vi "信息采集.vi"() -> (11 "Boolean":bool)   [LabVIEW 2023]
uses:
  <vilib>/sound2/lvsound2.llb/Sampling Mode.ctl
  <vilib>/sound2/lvsound2.llb/Sound Data Format.ctl
  <vilib>/sound2/lvsound2.llb/Sound Input Read (DBL).vi
panel:
  in  "退出信息采集":bool
  in  "Tab Control":enum32{"语音文字录入", "图片录入"}(tab)
  out "时间":string
  in  "保存语音文字信息":bool
  in  "开始录入语音":bool
  in  "停止录入语音":bool
  out "语音录入波形":waveform(dbl)[](graph)
  out "采集语音录入时间":string
  in  "Cluster":T1
  in  "图片录入":bool
  out "图片显示":picture
  # "个人信息采集"
  # "个人信息采集"
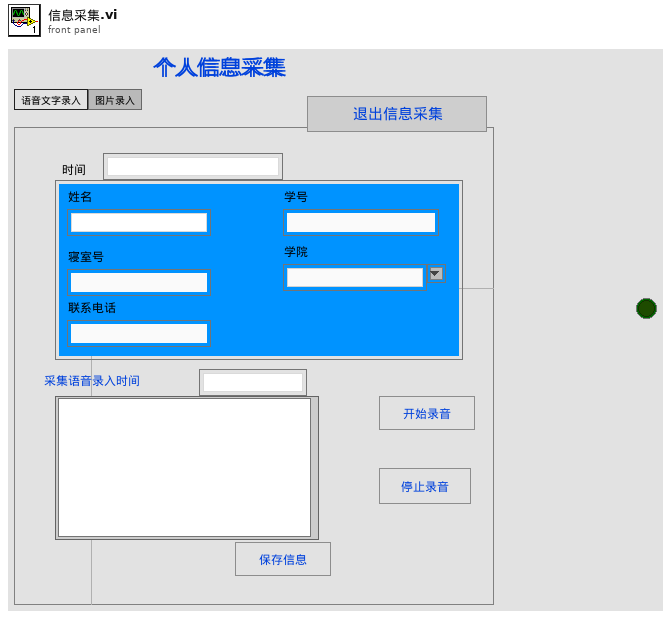
[diagram p1: front panel]
types:
  T1 = cluster{"学号":string, "姓名":string, "寝室号":string, "学院":string, "联系电话":string}
  T2 = typedef "Sound Data Format.ctl" = cluster{"sample rate (S/s)":dbl, "number of channels":i32, "bits per sample":i32}
  T3 = enum16{"open", "replace", "create", "open or create", "replace or create", "replace or create with confirmation"}
  T4 = typedef "Sampling Mode.ctl" = i32
  T5 = typedef "Sound Input Task ID.ctl" = u32
  T6 = typedef "imagedata.ctl" = cluster{"image type":i32, "image depth":i32, "image":u8[], "mask":u8[], "colors":u32[], "Rectangle":cluster{"left":i16, "top":i16, "right":i16, "bottom":i16}}
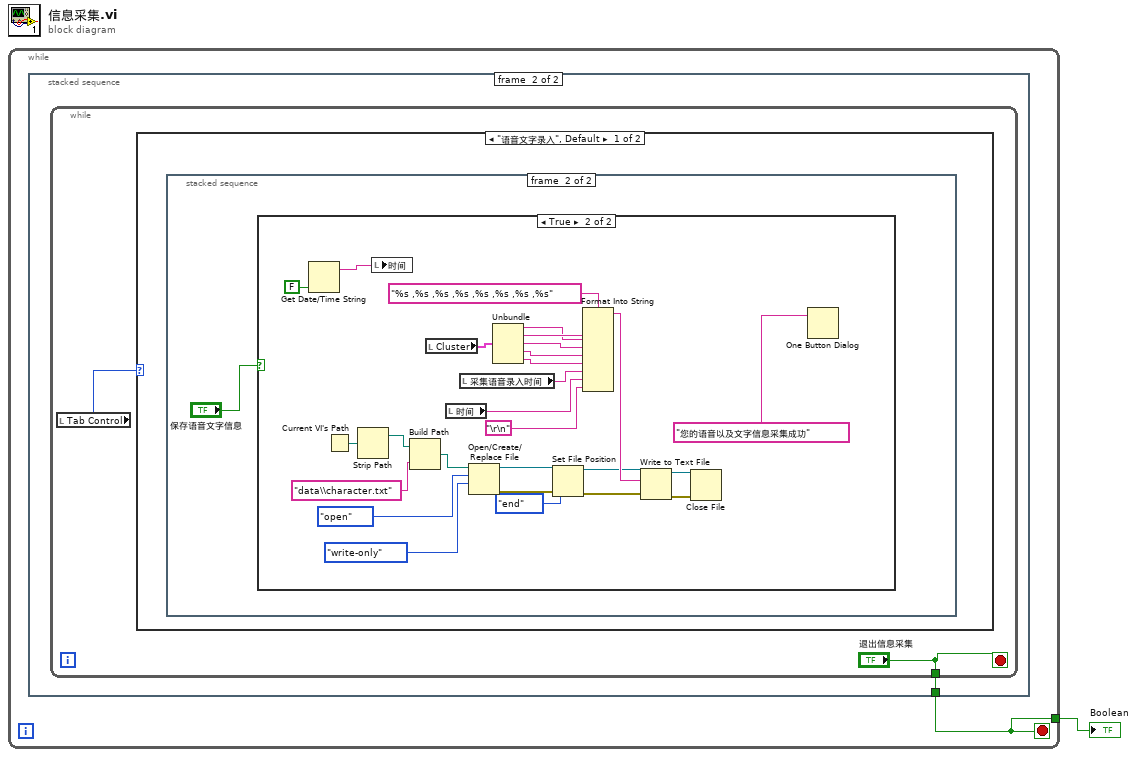
[diagram p0: block diagram]
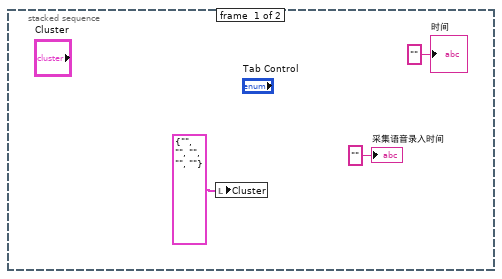
[diagram p2: hidden frame]
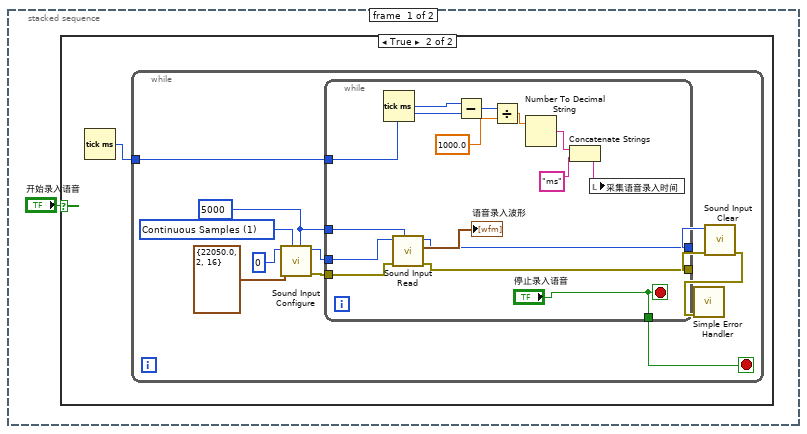
[diagram p3: hidden frame]
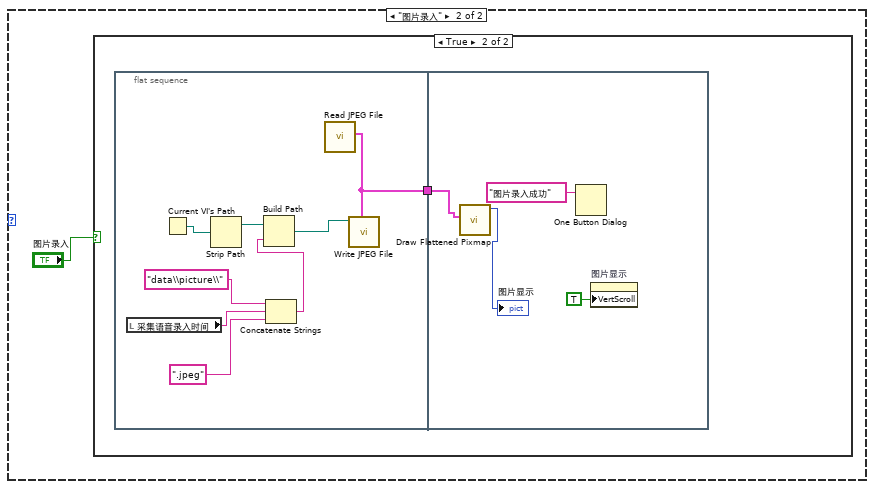
[diagram p6: hidden frame]
diagram:
  n1 = while {
    tunnel: [w2] -> w1
    stop <- w2 stop-if-true
    n2 = stacked-sequence {
      tunnel: [_ w6] -> w2
      frame #0 {
        n3 = local write "Cluster"(T1 {"学号"="", "姓名"="", "寝室号"="", "学院"="", "联系电话"=""} ("Cluster")) -> ()
        "时间" <- "" ("录入时间")
        "采集语音录入时间" <- "" ("语音录入时间")
      }
      frame #1 {
        n4 = while {
          tunnel: ["退出信息采集"] -> w6
          stop <- "退出信息采集" stop-if-true
          n5 = local read "Tab Control"() -> (w8:enum32{"语音文字录入", "图片录入"})
          n6 = case shown="\"语音文字录入\", Default" w8 {
            frame "语音文字录入", Default {
              n7 = stacked-sequence {
                frame #0 {
                  n8 = case shown="True" "开始录入语音" {
                    frame False {
                    }
                    frame True {
                      n9 = Tick Count (ms)() -> (millisecond timer value=w10:u32)
                      n10 = while {
                        tunnel: w10 -> [w12]
                        stop <- w11 stop-if-true
                        w19 = 5000 ("number of samples/ch")
                        w21 = T4 1 items=["Finite Samples", "Continuous Samples"] ("sample mode")
                        n11 = call <vilib>:"Sound Input Configure.vi"("number of samples/ch"=w19, "sample mode"=w21, "sound format"=T2 {"sample rate (S/s)"=22050.0, "number of channels"=2, "bits per sample"=16}, "device ID"=u32 0) -> ("error out"=w16:errorcluster, "task ID"=w17:T5)  [unwired: 6 in]
                        n12 = while {
                          tunnel: w19 -> [w36]
                          tunnel: w17 -> [w35]
                          tunnel: w16 -> [w34]
                          tunnel: [w32] -> w15
                          tunnel: [w31] -> w14
                          tunnel: w12 -> [w29]
                          tunnel: ["停止录入语音"] -> w11
                          stop <- "停止录入语音" stop-if-true
                          n13 = Tick Count (ms)() -> (millisecond timer value=w30:u32)
                          n14 = call-poly <vilib>:"Sound Input Read.vi"("number of samples/ch"=w36, "error in (no error)"=w34, "task ID"=w35) -> ("error out"=w31:errorcluster, "data"=→"语音录入波形":waveform(dbl)[], "task ID out"=w32:T5)  [unwired: 6 in]
                          n15 = Subtract(x=w30, y=w29) -> (x-y=w27:u32)
                          n16 = Divide(x=w27, y=1000.0) -> (x/y=w26:dbl)
                          n17 = Number To Decimal String(number=w26) -> (decimal integer string=w25:string)  [unwired: 1 in]
                          n18 = Concatenate Strings(w25, "ms" ("string")) -> (w23:string)
                          n19 = local write "采集语音录入时间"(w23) -> ()
                        }
                        n20 = call <vilib>:"Sound Input Clear.vi"("error in (no error)"=w14, "task ID"=w15) -> ("error out"=w13:errorcluster)  [unwired: 9 in]
                        n21 = call <vilib>:"Simple Error Handler.vi"("error in (no error)"=w13) -> ()  [unwired: 4 in, 5 out]
                      }
                    }
                  }
                }
                frame #1 {
                  n22 = case shown="True" "保存语音文字信息" {
                    frame False {
                    }
                    frame True {
                      n23 = Get Date/Time String(want seconds? (F)=FALSE) -> (date string=w56:string)  [unwired: 2 in, 1 out]
                      n24 = Current VI's Path() -> (path=w55:path)
                      n25 = Strip Path(path=w55) -> (stripped path=w54:path)  [unwired: 1 out]
                      n26 = local write "时间"(w56) -> ()
                      n27 = Build Path(base path=w54, name or relative path="data\\character.txt") -> (appended path=w50:path)
                      n28 = local read "Cluster"() -> (w64:T1)
                      n29 = local read "时间"() -> (w52:string)
                      n30 = local read "采集语音录入时间"() -> (w53:string)
                      n31 = Open/Create/Replace File(file path (use dialog)=w50, operation (0:open)=T3."open", access (0:read/write)=enum16{"read/write", "read-only", "write-only"}."write-only") -> (refnum out=w42:refnum<file>, error out=w40:errorcluster)  [unwired: 3 in, 1 out]
                      n32 = Unbundle(w64) -> ("学号"=w61:string, "姓名"=w62:string, "寝室号"=w60:string, "学院"=w59:string, "联系电话"=w58:string)
                      n33 = Set File Position(refnum=w42, from (0:start)=enum16{"start", "end", "current"}."end", error in=w40) -> (refnum out=w41:refnum<file>, error out=w39:errorcluster)  [unwired: 1 in]
                      n34 = Format Into String(format string="%s ,%s ,%s ,%s ,%s ,%s ,%s ,%s", w62, w61, w60, w59, w58, w53, w52, "\r\n") -> (resulting string=w46:string)  [unwired: 2 in, 1 out]
                      n35 = Write to Text File(file (use dialog)=w41, text=w46, error in=w39) -> (refnum out=w44:refnum<file>, error out=w45:errorcluster)  [unwired: 1 in, 1 out]
                      n36 = Close File(refnum=w44, error in=w45) -> ()  [unwired: 2 out]
                      n37 = One Button Dialog(message="您的语音以及文字信息采集成功") -> ()  [unwired: 1 in, 1 out]
                    }
                  }
                }
              }
            }
            frame "图片录入" {
              n38 = case shown="True" "图片录入" {
                frame False {
                }
                frame True {
                  n39 = flat-sequence {
                    tunnel: [w67] -> w66
                    tunnel: w66 -> [w78]
                    frame #0 {
                      n40 = local read "采集语音录入时间"() -> (w70:string)
                      n41 = Current VI's Path() -> (path=w74:path)
                      n42 = Strip Path(path=w74) -> (stripped path=w73:path)  [unwired: 1 out]
                      n43 = Concatenate Strings("data\\picture\\" ("string"), w70, ".jpeg" ("string")) -> (w69:string)
                      n44 = Build Path(base path=w73, name or relative path=w69) -> (appended path=w68:path)
                      n45 = call <vilib>:"Read JPEG File.vi"() -> ("image data"=w67:T6)  [unwired: 9 in, 2 out]
                      n46 = call <vilib>:"Write JPEG File.vi"("image data"=w67, "path to JPEG file"=w68) -> ()  [unwired: 8 in, 2 out]
                    }
                    frame #1 {
                      n47 = call <vilib>:"Draw Flattened Pixmap.vi"("image data"=w78) -> ("new picture"=→"图片显示":picture)  [unwired: 8 in]
                      n48 = One Button Dialog(message="图片录入成功") -> ()  [unwired: 1 in, 1 out]
                      n49 = property on="图片显示" class="Pict"("VertScroll"=TRUE ("Vertical Scrollbar Visible")) -> ()  [unwired: 2 in, 2 out]
                    }
                  }
                }
              }
            }
          }
        }
      }
    }
  }
  "Boolean" <- w1
